vi "BroadcastConnectionStatus.vi"(8 "error in (no error)":errorcluster, 10 "status":T1, 11 "Qbus in":refnum<class "Qbus.lvclass">) -> (0 "error out":errorcluster, 3 "Qbus out":refnum<class "Qbus.lvclass">)   [LabVIEW 2017, in "ServerComm.lvlib"]
uses:
  <vilib>/addons/InsightCM/Devices/Shared/Common/ServerComm/ServerComm.lvlib
  <vilib>/addons/Qbus/Qbus.lvclass
  <vilib>/addons/InsightCM/Devices/Shared/Common/ServerComm/controls/ConnectionStatus.ctl
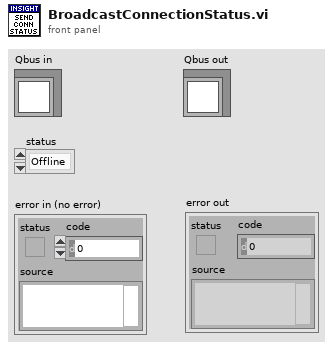
[diagram p1: front panel]
types:
  T1 = typedef "ServerComm.lvlib/ConnectionStatus.ctl" = enum16{"Offline", "NotAuthorized", "Online"}
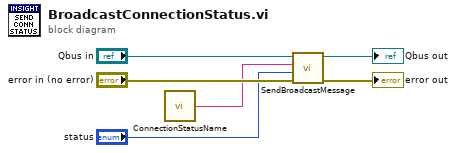
[diagram p0: block diagram]
diagram:
  n1 = call <vilib>:"ConnectionStatusName.vi"() -> ("message name"=w1:string)  [unwired: 5 in]
  n2 = call <vilib>:"SendBroadcastMessage.vi"("error in (no error)"="error in (no error)", "message value"="status", "message name"=w1, "Qbus in"="Qbus in") -> ("error in (no error)"=→"error out":errorcluster, "Qbus out"=→"Qbus out":refnum<class "Qbus.lvclass">)  [unwired: 6 in]
